vi "solar Find (Target).vi"(9 "Target":string, 10 "Targets":T1[](array[typedef])) -> (1 "Target Index":i32, 2 "Target Names":string[](array[string]))   [LabVIEW 2018]
doc: "This funds the target by name. The 'MAIN' target returns the top level target index."
uses:
  solar_ctl Target Global.ctl
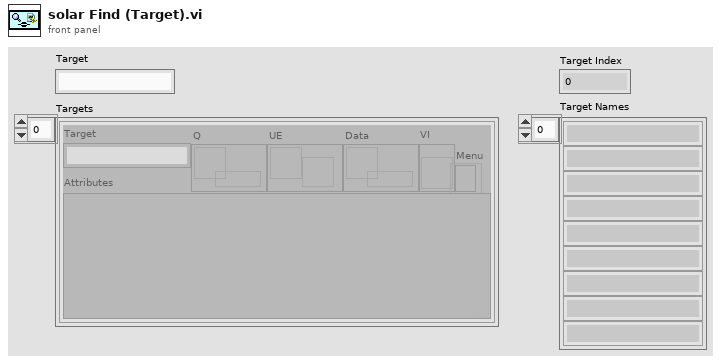
[diagram p1: front panel]
types:
  T1 = typedef "solar_ctl Target Global.ctl" = cluster{"Target":string, "Q":refnum<queue>, "UE":refnum<user-event>, "VI":refnum<vi>, "Menu":refnum<k9>, "Data":refnum<data-value>, "Attributes":variant}
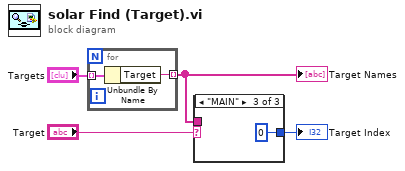
[diagram p0: block diagram]
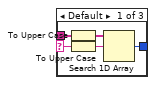
[diagram p2: hidden frame]
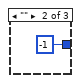
[diagram p3: hidden frame]
diagram:
  n1 = for {
    tunnel: [w6] -> w2 mode=indexing
    tunnel: "Targets" -> [w5] mode=indexing
    n2 = Unbundle By Name(w5) -> ("Target"=w6:string)
  }
  "Target Names" <- w2
  n3 = case shown="\"MAIN\"" "Target" {
    selector: "Target" -> [w7 _ _]
    tunnel: w2 -> [w11 _ _]
    tunnel: [w8 -1 ("index of element") 0 ("index of element")] -> w4
    frame Default {
      n4 = To Upper Case(1:w11) -> (0:w10:string[])
      n5 = To Upper Case(1:w7) -> (0:w9:string)
      n6 = Search 1D Array(1D array=w10, element=w9) -> (index of element=w8:i32)  [unwired: 1 in]
    }
    frame "" {
    }
    frame "MAIN" {
    }
  }
  "Target Index" <- w4
